vi "Do.vi"(8 "error in (no error)":errorcluster, 10 "Actor in":refnum<class "Actor.lvclass">, 11 "Terminate Sequencer Msg":refnum<class "Batch Msg.lvclass">) -> (0 "error out":errorcluster, 2 "Actor out":refnum<class "Actor.lvclass">)   [LabVIEW 2020, in "Sequencer.lvlib" / "Batch Msg.lvclass"]
doc: "Enqueue the message array in front on the Sequencer Core."
uses:
  Batch Msg.lvclass
  C:/Current projects/WS/Framework/Framework/Actors/Sequencer/Sequencer Messages/Sequencer Msg/Sequencer Msg.lvclass
  PPL/HDH.Actor Framework.Core.Actor.lvlibp/1abvi3w/vi.lib/ActorFramework/Actor/Actor.lvclass
  Sequencer/Sequencer.lvclass
  C:/Current projects/WS/PPL/HDH.Actor Framework.Core.Actor.lvlibp/1abvi3w/vi.lib/ActorFramework/Actor/Actor.lvclass
  Sequencer Msg/Sequencer Msg.lvclass/Sequencer Msg.ctl
  Batch Msg.lvclass/Batch Msg.ctl
  Sequencer Msg/Sequencer Msg.lvclass
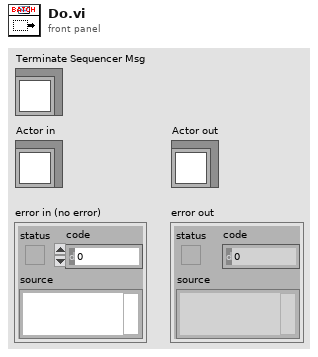
[diagram p1: front panel]
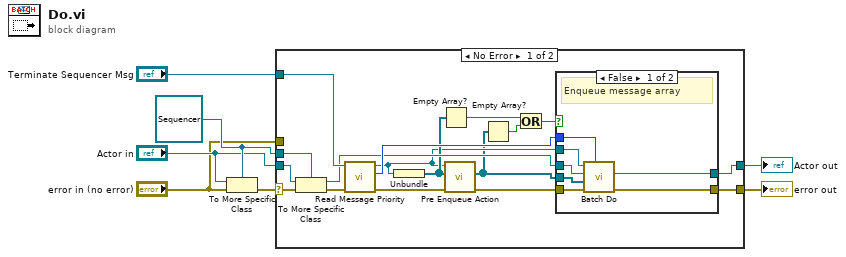
[diagram p0: block diagram]
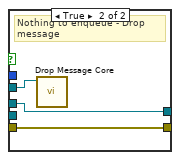
[diagram p2: hidden frame]
diagram:
  w5 = refnum<class "Sequencer.lvclass"> refnum ("Sequencer.lvlib:Sequencer.lvclass")
  n1 = To More Specific Class(target class=w5, reference="Actor in", error in="error in (no error)") -> (error out=w6:errorcluster)  [unwired: 1 out]
  n2 = case shown="No Error" w6 {
    selector: w6 -> [w21 _]
    tunnel: "Terminate Sequencer Msg" -> [w24 _]
    tunnel: w5 -> [w22 _]
    tunnel: "Actor in" -> [w20 w35]
    tunnel: [w18 w35] -> w3
    tunnel: [w17 w36] -> w2
    tunnel: "error in (no error)" -> [_ w36]
    frame No Error {
      n3 = To More Specific Class(target class=w22, reference=w20, error in=w21) -> (specific class reference=w19:refnum<class "Sequencer.lvclass">, error out=w16:errorcluster)
      n4 = call "Read Message Priority.vi"("error in (no error)"=w16, "Sequencer Msg in"=w24) -> ("error out"=w15:errorcluster, "Priority"=w23:u16, "Sequencer Msg out"=w11:refnum<class "Batch Msg.lvclass">)  [unwired: 7 in]
      n5 = Unbundle(w11) -> (w12:refnum<class "Message.lvclass">[])
      n6 = Empty Array?(array=w12) -> (empty?=w13:bool)
      n7 = call-dynamic "Pre Enqueue Action.vi"("error in (no error)"=w15, "Message Array in"=w12, "Msg in"=w11) -> ("error out"=w14:errorcluster, "Message Array out"=w10:refnum<class "Message.lvclass">[])  [unwired: 7 in]
      n8 = Empty Array?(array=w10) -> (empty?=w8:bool)
      n9 = Or(x=w13, y=w8) -> (x .or. y?=w9:bool)
      n10 = case "Enqueue if not empty" shown="False" w9 {
        tunnel: w23 -> [w25 _]
        tunnel: w19 -> [w27 w34]
        tunnel: [w26 w34] -> w18
        tunnel: [w31 w33] -> w17
        tunnel: w14 -> [w30 w33]
        tunnel: w10 -> [w28 _]
        tunnel: w11 -> [w29 w32]
        frame False {
          # "Enqueue message array"
          n11 = call-dynamic "Batch Do.vi"("Priority"=w25, "error in (no error)"=w30, "Message Array in"=w28, "Sequencer in"=w27, "Batch Msg"=w29) -> ("error out"=w31:errorcluster, "Sequencer out"=w26:refnum<class "Sequencer.lvclass">)  [unwired: 5 in]
        }
        frame True {
          # "Nothing to enqueue - Drop message"
          n12 = call-dynamic "Drop Message Core.vi"("Message in"=w32) -> ()  [unwired: 11 in]
        }
      }
    }
    frame Error {
    }
  }
  "error out" <- w2
  "Actor out" <- w3
